vi "Fittinglogistic_MODCA.vi"(9 "Paramter guess":dbl[](array[numeric])=[-4.2, 0.0, 100.0, 1.0, 1.0], 10 "y":dbl[](array[numeric]), 11 "t":dbl[](array[numeric])) -> (0 "fitting (y&T)":dbl[][](array[numeric]), 1 "E":i32, 2 "XY Graph":cluster{cdb[]}[](graph), 3 "output cluster":T1)   [LabVIEW 2014]
uses:
  <vilib>/gmath/NI_Gmath.lvlib
  <vilib>/gmath/NumericalOptimization/Nonlinear Curve Fit LM.vi
panel:
  out "x0":dbl
  out "fit curve":T2(graph)
  out "y0":dbl
  out "slope":cluster{"all rows":dbl[], dbl[]}(graph)
  out "best fit parameters":dbl[](array[numeric])
  out "error out":errorcluster
  # "y0"
  # "x0"
  # "k"
  # "L"
  # "a"
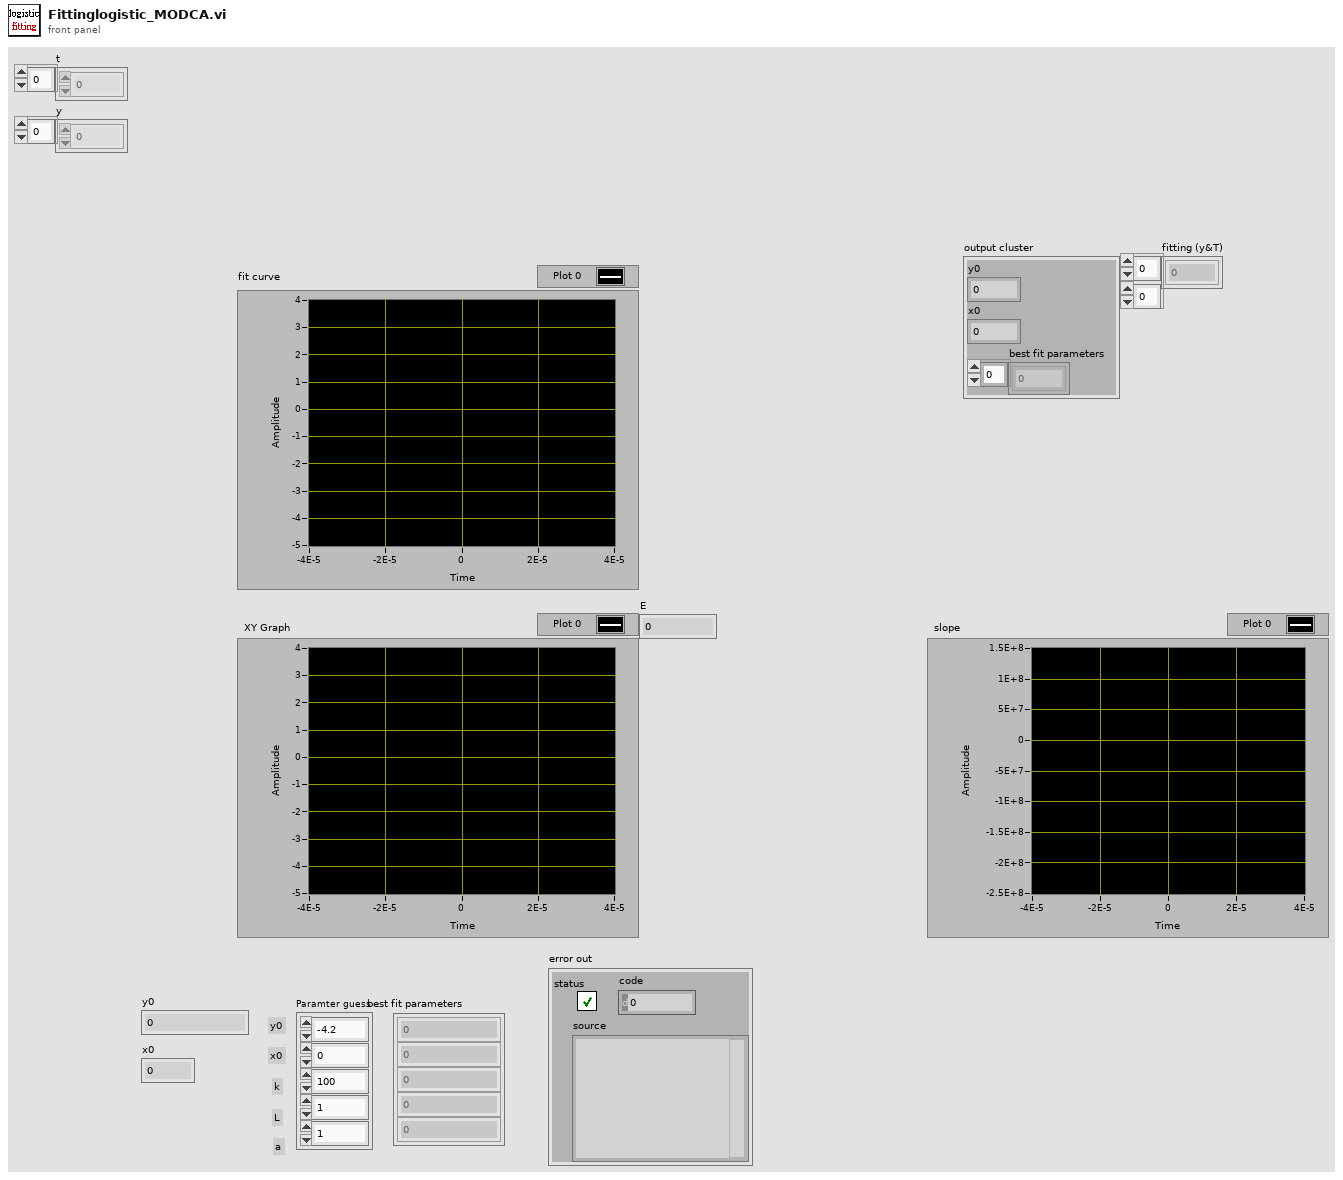
[diagram p1: front panel]
types:
  T1 = cluster{"y0":dbl, "x0":dbl, "best fit parameters":dbl[]}
  T2 = cluster{"all rows":dbl[], "best nonlinear fit":dbl[]}
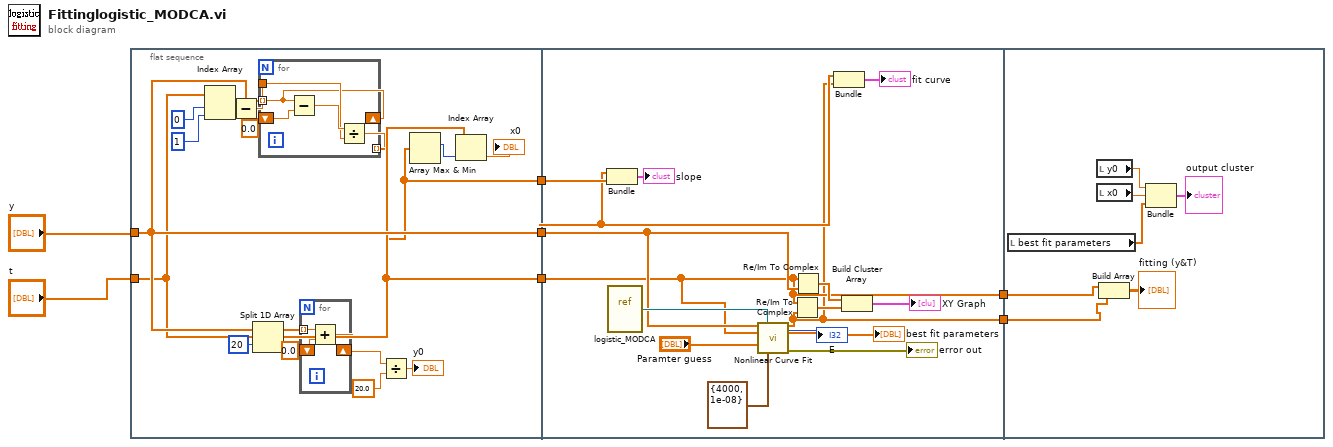
[diagram p0: block diagram]
diagram:
  n1 = flat-sequence {
    tunnel: "y" -> [w14]
    tunnel: "t" -> [w13]
    tunnel: [w10] -> w7
    tunnel: [w13] -> w6
    tunnel: [w14] -> w5
    tunnel: w7 -> [w37]
    tunnel: w6 -> [w34]
    tunnel: w5 -> [w36]
    tunnel: [w34] -> w2
    tunnel: [w33] -> w1
    tunnel: w2 -> [w50]
    tunnel: w1 -> [w49]
    frame #0 {
      n2 = Index Array(array=w13, index #1=0 ("index"), index #2=1 ("index")) -> (element #1=w20:dbl, element #2=w19:dbl)
      n3 = Subtract(x=w19, y=w20) -> (x-y=w21:dbl)
      n4 = Split 1D Array(array=w14, index=20) -> (first subarray=w22:dbl[])  [unwired: 1 out]
      n5 = for {
        shift-right: [w28] -> _
        shift-left: 0.0 ("Numeric") -> [w32]
        tunnel: w14 -> [w28] mode=indexing
        tunnel: w21 -> [w30]
        tunnel: [w29] -> w10 mode=indexing
        n6 = Subtract(x=w28, y=w32) -> (x-y=w31:dbl)
        n7 = Divide(x=w31, y=w30) -> (x/y=w29:dbl)
      }
      n8 = for {
        tunnel: w22 -> [w25] mode=indexing
        shift-right: [w27] -> w23
        shift-left: 0.0 -> [w26]
        n9 = Add(x=w25, y=w26) -> (x+y=w27:dbl)
      }
      n10 = Divide(x=w23, y=20.0) -> (x/y=→"y0":dbl)
      n11 = Array Max & Min(array=w10) -> (max index (indices)=w24:i32)  [unwired: 3 out]
      n12 = Index Array(array=w13, index=w24) -> (element=→"x0":dbl)
    }
    frame #1 {
      n13 = Bundle("t"=w34, w37) -> (→"slope":cluster{"t":dbl[], dbl[]})  [unwired: 1 in]
      n14 = vi-ref "logistic_MODCA.vi"() -> (w43:refnum<vi>)
      n15 = call-poly <vilib>:"Nonlinear Curve Fit.vi"("Y"=w36, "f(x,a)"=w43, "X"=w34, "initial parameters"="Paramter guess", "termination"=cluster{"max iteration":i32, "tolerance":dbl} {"max iteration"=4000, "tolerance"=1e-08}) -> ("number of function calls"=→"E":i32, "best nonlinear fit"=w33:dbl[], "best fit parameters"=→"best fit parameters":dbl[], "error out"=→"error out":errorcluster)  [unwired: 5 in, 2 out]
      n16 = Re/Im To Complex(1:w33, 2:w34) -> (0:w46:cdb[])
      n17 = Re/Im To Complex(1:w36, 2:w34) -> (0:w47:cdb[])
      n18 = Bundle("t"=w34, "best nonlinear fit"=w33) -> (→"fit curve":cluster{"t":dbl[], "best nonlinear fit":dbl[]})  [unwired: 1 in]
      n19 = Build Cluster Array(w47, w46) -> (→"XY Graph":cluster{cdb[]}[])
    }
    frame #2 {
      n20 = local read "best fit parameters"() -> (w52:dbl[])
      n21 = local read "y0"() -> (w54:dbl)
      n22 = local read "x0"() -> (w53:dbl)
      n23 = Build Array(w50, w49) -> (→"fitting (y&T)":dbl[][])
      n24 = Bundle("y0"=w54, "x0"=w53, "best fit parameters"=w52) -> (→"output cluster":T1)  [unwired: 1 in]
    }
  }
